vi "Beam_Check_Positions.vi"(0 "Load From File?":bool, 7 "Give Focal Point Info (F)":bool, 11 "Primary Positions In":dbl[][](array[numeric])) -> (1 "Fixed Axis":T1, 2 "More Info":string[][](array[string]), 3 "Setup File":string[](array[string]), 4 "Beam Info":T2(array[cluster]), 6 "Beam Names":string[](array[string]), 10 "Primary Beam Positions":dbl[][](array[numeric]), 12 "Focal Length":dbl[](array[numeric]), 14 "Wavelength (nm)":dbl[](array[numeric]), 15 "Power (mW)":dbl[](array[numeric]))   [LabVIEW 2020]
uses:
  Controls/Fixed Axis.ctl
  Globals/Meas_global.vi
  Globals/Constants_global.vi
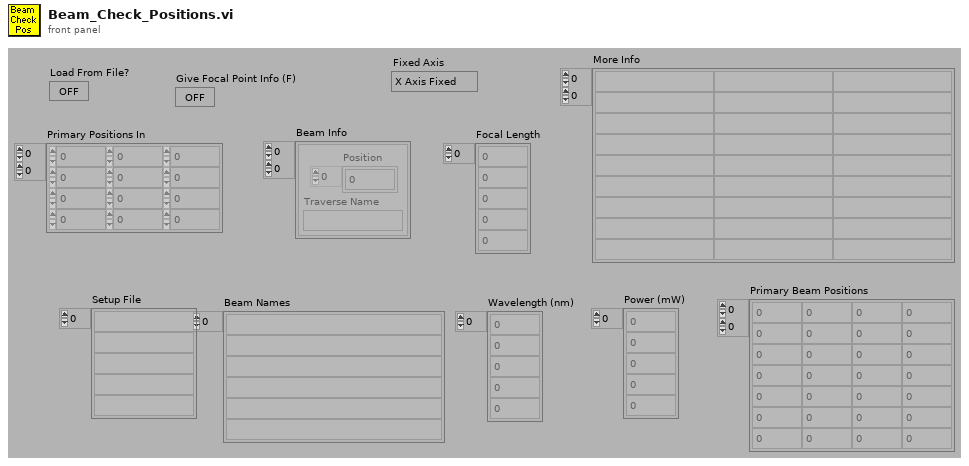
[diagram p1: front panel]
types:
  T1 = typedef "Fixed Axis.ctl" = enum16{"X Axis Fixed", "Y Axis Fixed", "Z Axis Fixed"}
  T2 = cluster{"Position":dbl[], "Traverse Name":string}[][]
  T3 = typedef "Post_Process.ctl" = enum16{"Take New Data", "Post Process Raw Data File"}
  T4 = cluster{"Position":dbl[], "Traverse Name":string}
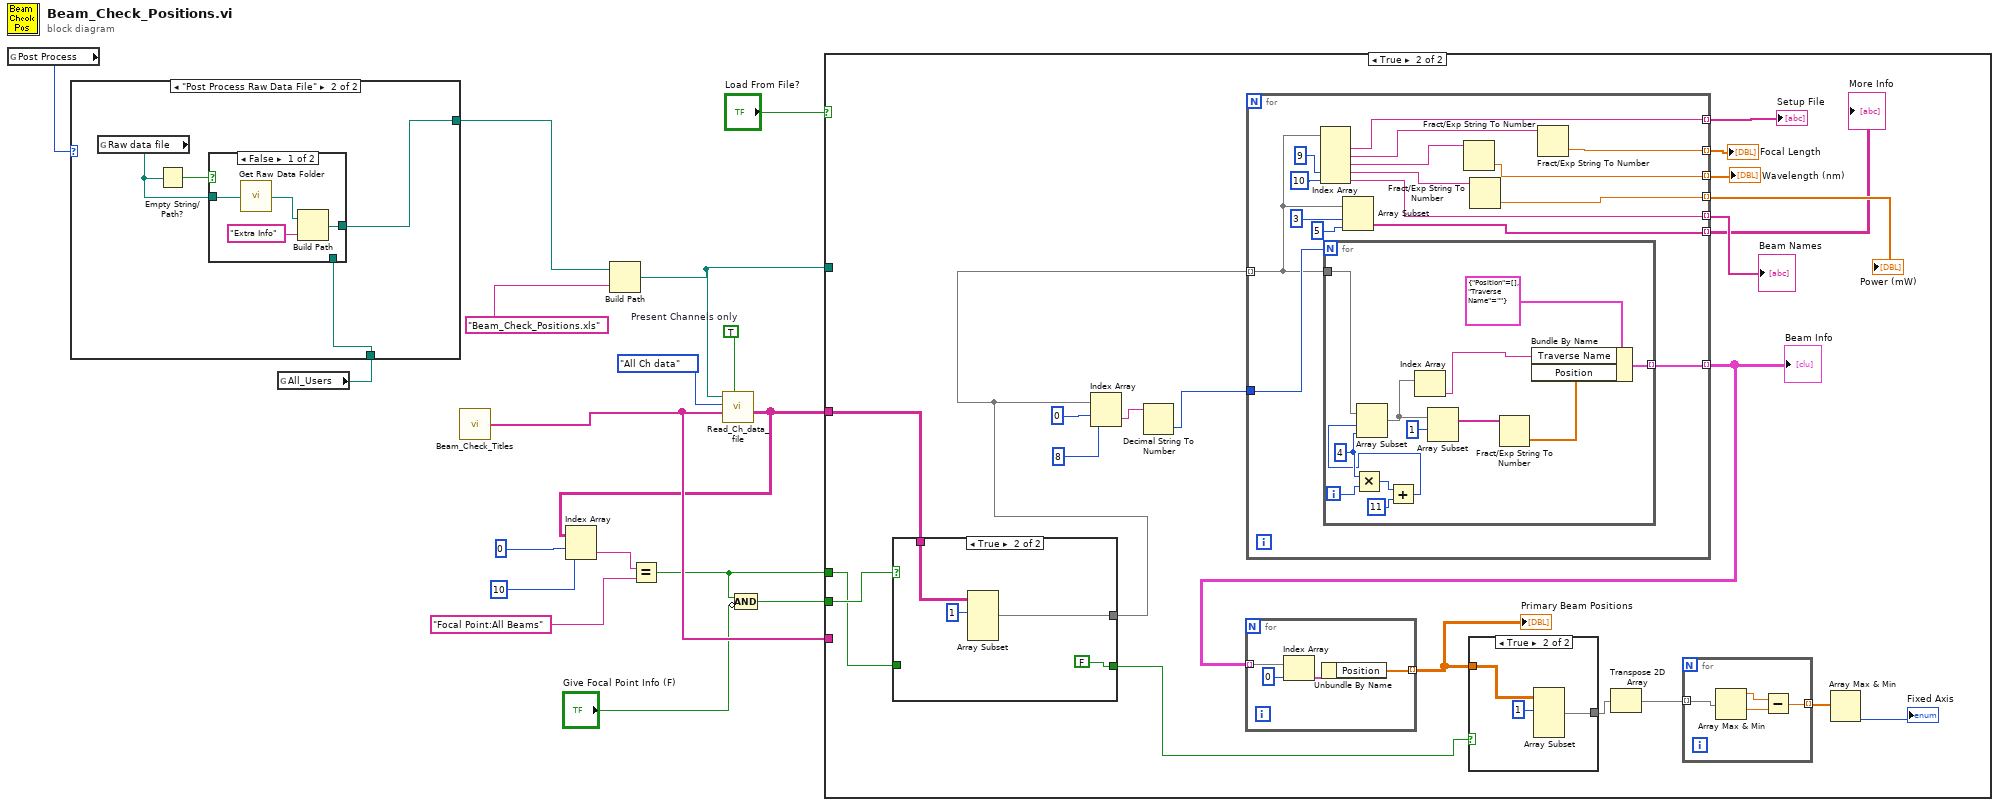
[diagram p0: block diagram]
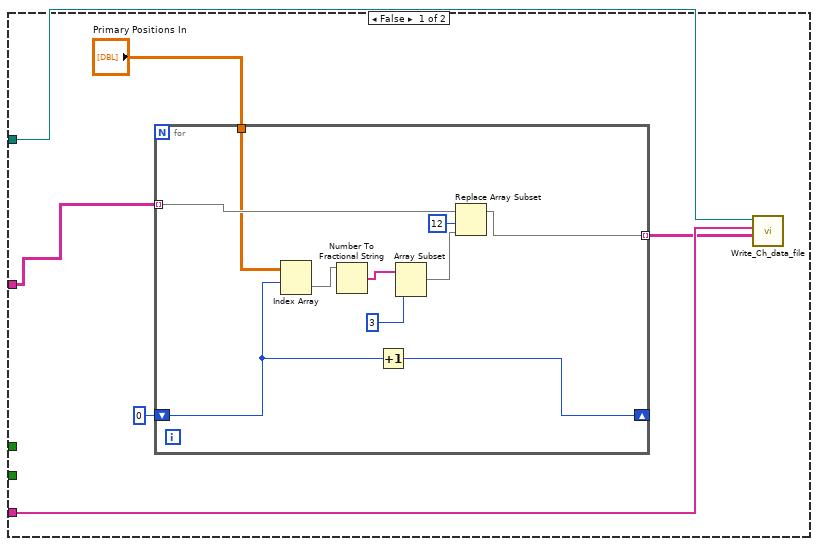
[diagram p4: hidden frame]
diagram:
  w16 = TRUE  # Present Channels only
  n1 = global read "Meas_global.vi" "Post Process"() -> (w1:T3)
  n2 = global read "Constants_global.vi" "All_Users"() -> (w3:path)
  n3 = case shown="\"Post Process Raw Data File\"" w1 {
    tunnel: [w18 w22] -> w2
    tunnel: w3 -> [w18 w19]
    frame "Take New Data" {
    }
    frame "Post Process Raw Data File" {
      n4 = global read "Meas_global.vi" "Raw data file"() -> (w21:path)
      n5 = Empty String/Path?(string/path=w21) -> (empty?=w20:bool)
      n6 = case shown="False" w20 {
        tunnel: [w23 w27] -> w22
        tunnel: w21 -> [w26 _]
        tunnel: w19 -> [_ w27]
        frame False {
          n7 = call "Get Raw Data Folder.vi"("Raw data file"=w26) -> ("Main Raw Data Folder"=w24:path)
          n8 = Build Path(base path=w24, name or relative path="Extra Info") -> (appended path=w23:path)
        }
        frame True {
        }
      }
    }
  }
  n9 = call "Beam_Check_Titles.vi"() -> ("Titles"=w12:string[])
  n10 = Build Path(base path=w2, name or relative path="Beam_Check_Positions.xls" ("Substring")) -> (appended path=w13:path)
  n11 = call "Read_Ch_data_file.vi"("Present Channels only"=w16, "Present Channels"=w12, "Output"=enum16{"All Ch data", "The last few rows"}."All Ch data", "Filename"=w13) -> ("Channel Values"=w9:string[][])  [unwired: 1 in, 4 out]
  n12 = Index Array(array=w9, index (row)=0, index (col)=10 ("disabled index (col)")) -> (element=w8:string)
  n13 = Equal?(x=w8, y="Focal Point:All Beams") -> (x = y?=w4:bool)
  n14 = Compound Arithmetic op=AND(w4, invert "Give Focal Point Info (F)") -> (w5:bool)
  n15 = case shown="True" "Load From File?" {
    tunnel: w9 -> [w33 w56]
    tunnel: w13 -> [w31 _]
    tunnel: w12 -> [w30 _]
    tunnel: w5 -> [_ w55]
    tunnel: w4 -> [_ w48]
    frame False {
      n16 = for {
        tunnel: w33 -> [w43] mode=indexing
        tunnel: "Primary Positions In" -> [w42]
        tunnel: [w41] -> w29 mode=indexing
        shift-right: [w40] -> _
        shift-left: 0 -> [w39]
        n17 = Index Array(array=w42, index (row)=w39) -> (element=w34:dbl[])  [unwired: 1 in]
        n18 = Number To Fractional String(number=w34) -> (F-format string=w37:string[])  [unwired: 3 in]
        n19 = Increment(x=w39) -> (x+1=w40:i32)
        n20 = Array Subset(array=w37, length=3) -> (w35:string[])  [unwired: 1 in]
        n21 = Replace Array Subset(array=w43, new element=w35, index=12) -> (w41:string[])
      }
      n22 = call "Write_Ch_data_file.vi"("Channel Values"=w29, "Channel names"=w30, "Filename"=w31) -> ()  [unwired: 4 in, 5 out]
    }
    frame True {
      n23 = case shown="True" w55 {
        tunnel: w56 -> [w74 w78]
        tunnel: [w74 w76] -> w54
        tunnel: w48 -> [w73 _]
        tunnel: [w73 FALSE] -> w47
        frame False {
        }
        frame True {
          n24 = Array Subset(array=w78, index (row)=1 ("index")) -> (w76:string[][])  [unwired: 3 in]
        }
      }
      n25 = Index Array(array=w54, index (row)=0, index (col)=8 ("disabled index (col)")) -> (element=w62:string)
      n26 = Decimal String To Number(string=w62) -> (number=w61:i32)  [unwired: 2 in, 1 out]
      n27 = for {
        tunnel: w54 -> [w86] mode=indexing
        tunnel: w61 -> [w98]
        tunnel: [w97] -> w60 mode=indexing
        tunnel: [w90] -> w59 mode=indexing
        tunnel: [w96] -> w58 mode=indexing
        tunnel: [w93] -> w57 mode=indexing
        tunnel: [w95] -> w52 mode=indexing
        tunnel: [w94] -> w53 mode=indexing
        tunnel: [w83] -> w44 mode=indexing
        n28 = Index Array(array=w86, index #4=9 ("index"), index #5=10 ("index")) -> (element #1=w93:string, element #2=w92:string, element #3=w91:string, element #4=w87:string, element #5=w90:string)  [unwired: 3 in]
        n29 = for {
          N: w98 -> [_]
          tunnel: w86 -> [w111]
          tunnel: [w104] -> w97 mode=indexing
          i -> [w109]
          w110 = 4 ("length")
          n30 = Multiply(x=w110, y=w109) -> (x*y=w108:i32)
          n31 = Add(x=w108, y=11) -> (x+y=w106:i32)
          n32 = Array Subset(array=w111, index=w106, length=w110) -> (w102:string[])
          n33 = Index Array(array=w102) -> (element=w105:string)  [unwired: 1 in]
          n34 = Array Subset(array=w102, index=1) -> (w100:string[])  [unwired: 1 in]
          n35 = Fract/Exp String To Number(string=w100) -> (number=w99:dbl[])  [unwired: 3 in, 1 out]
          n36 = Bundle By Name(cluster=T4 {"Position"=[], "Traverse Name"=""} ("Cluster"), "Traverse Name"=w105, "Position"=w99) -> (w104:T4)
        }
        n37 = Array Subset(array=w86, index=3, length=5) -> (w83:string[])
        n38 = Fract/Exp String To Number(string=w91) -> (number=w94:dbl)  [unwired: 3 in, 1 out]
        n39 = Fract/Exp String To Number(string=w87) -> (number=w96:dbl)  [unwired: 3 in, 1 out]
        n40 = Fract/Exp String To Number(string=w92) -> (number=w95:dbl)  [unwired: 3 in, 1 out]
      }
      "Beam Info" <- w60
      "Beam Names" <- w59
      "Power (mW)" <- w58
      "Setup File" <- w57
      "Wavelength (nm)" <- w53
      "Focal Length" <- w52
      "More Info" <- w44
      n41 = for {
        tunnel: w60 -> [w82] mode=indexing
        tunnel: [w79] -> w46 mode=indexing
        n42 = Index Array(array=w82, index=0) -> (element=w80:T4)
        n43 = Unbundle By Name(w80) -> ("Position"=w79:dbl[])
      }
      "Primary Beam Positions" <- w46
      n44 = case shown="True" w47 {
        tunnel: w46 -> [w65 w67]
        tunnel: [w65 w66] -> w45
        frame False {
        }
        frame True {
          n45 = Array Subset(array=w67, index (row)=1 ("index")) -> (w66:dbl[][])  [unwired: 3 in]
        }
      }
      n46 = Transpose 2D Array(2D array=w45) -> (transposed array=w51:dbl[][])
      n47 = for {
        tunnel: w51 -> [w72] mode=indexing
        tunnel: [w69] -> w50 mode=indexing
        n48 = Array Max & Min(array=w72) -> (max value=w71:dbl, min value=w70:dbl)  [unwired: 2 out]
        n49 = Subtract(x=w71, y=w70) -> (x-y=w69:dbl)
      }
      n50 = Array Max & Min(array=w50) -> (min index (indices)=→"Fixed Axis":i32)  [unwired: 3 out]
    }
  }
